vi "ma_windowed FFT.vi"(8 "error in (no error)":errorcluster, 9 "window":T1=1 items=["Rectangle"=0, "Hanning"=1, "Hamming"=2, "Blackman-Harris"=3, "Exact Blackman"=4, "Blackman"=5, "Flat Top"=6, "4 Term B-Harris "=7, "7 Term B-Harris"=8, "Low Sidelobe"=9, "Blackman Nuttall"=11, "Triangle"=30, "Bartlett-Hanning"=31, "Bohman"=32, "Parzen"=33, "Welch"=34, "Kaiser"=60, "Dolph-Chebyshev"=61, "Gaussian"=62], 10 "window parameter":dbl=nan, 11 "time signal X":waveform(dbl)) -> (0 "error out":errorcluster, 2 "df":dbl, 3 "Sx":cdb[](array[numeric]))   [LabVIEW 2020, in "NI_MAPro.lvlib"]
doc: "Computes the frequency response and the coherence based on the input signals. Results are returned as <B>real part</B>, <B>imaginary part</B>, and <B>coherence</B>."
uses:
  NI_MAPro.lvlib
  windowTd.ctl
  NI_AALPro.lvlib
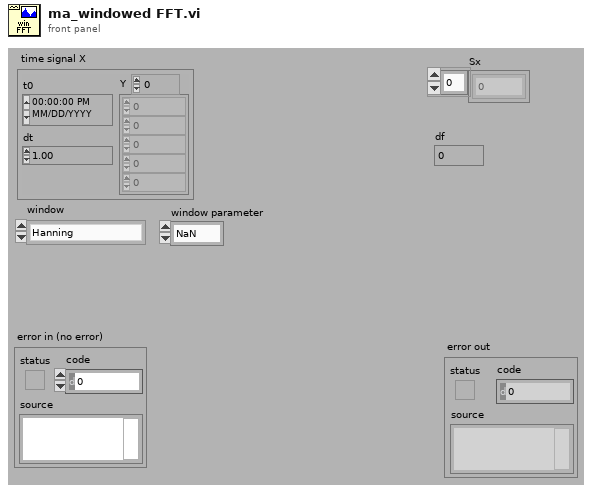
[diagram p1: front panel]
types:
  T1 = typedef "NI_AALPro.lvlib/windowTd.ctl" = u32
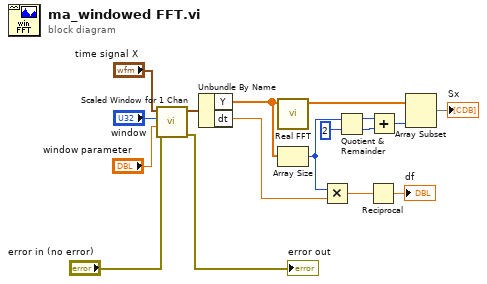
[diagram p0: block diagram]
diagram:
  n1 = call "Scaled Window for 1 Chan.vi"("error in (no error)"="error in (no error)", "window parameter"="window parameter", "window"="window", "signal in"="time signal X") -> ("error out"=→"error out":errorcluster, "signal out"=w15:waveform(dbl))  [unwired: 5 in, 1 out]
  n2 = Unbundle By Name(w15) -> ("Y"=w5:dbl[], "dt"=w3:dbl)
  n3 = call "Real FFT.vi"("X"=w5) -> ("FFT {X}"=w13:cdb[])  [unwired: 9 in, 1 out]
  n4 = Array Size(array=w5) -> (size(s)=w14:i32)
  n5 = Multiply(x=w14, y=w3) -> (x*y=w12:dbl)
  n6 = Quotient & Remainder(x=w14, y=2) -> (x-y*floor(x/y)=w10:i32, floor(x/y)=w9:i32)
  n7 = Reciprocal(x=w12) -> (1/x=→"df":dbl)
  n8 = Add(x=w10, y=w9) -> (x+y=w7:i32)
  n9 = Array Subset(array=w13, length=w7) -> (→"Sx":cdb[])  [unwired: 1 in]
